vi "S2C_UNITHERM_Proc_CacheState.vi"(7 "Label":string, 8 "Error In":errorcluster, 11 "Data In":string) -> (0 "Error Out":errorcluster, 3 "Data Out":string)   [LabVIEW 2024]
uses:
  S2C_UNITHERM_Proc_Globals.vi
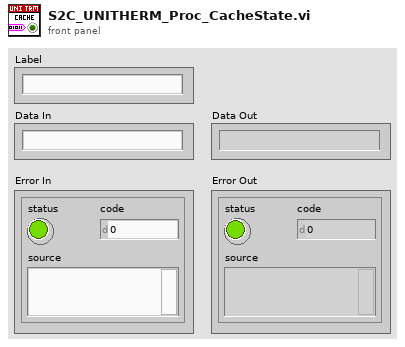
[diagram p1: front panel]
types:
  T1 = cluster{"Resource Name":string, "Baud Rate":u32, "Data Bits":u16, "Parity":u16, "Stop Bits":u16, "Flow Control":u16, "Termination Char":u8, "Enable Termination":bool, "Timeout":u32}
  T2 = cluster{"Resource Name":refnum<visa-resource-name>, "Baud Rate":u32, "Data Bits":u16, "Parity":u16, "Stop Bits":u16, "Flow Control":u16, "Termination Char":u8, "Enable Termination":bool, "Timeout":u32, "P1C1Exe":bool}
  T3 = cluster{"Command":string, "Action":string, "P2C1Exe":bool}
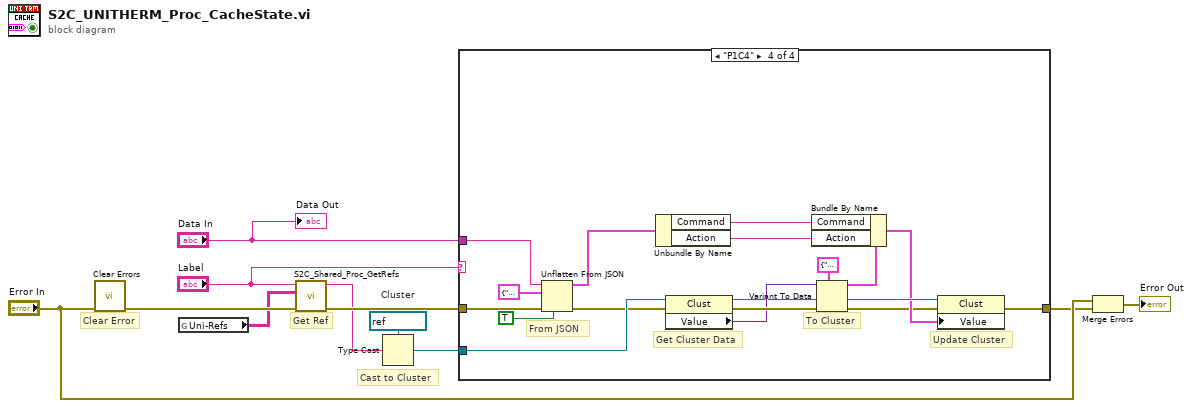
[diagram p0: block diagram]
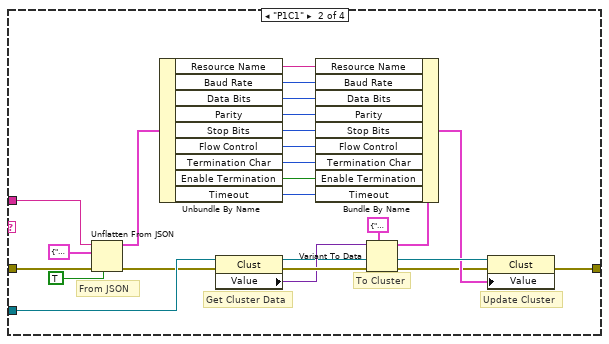
[diagram p3: hidden frame]
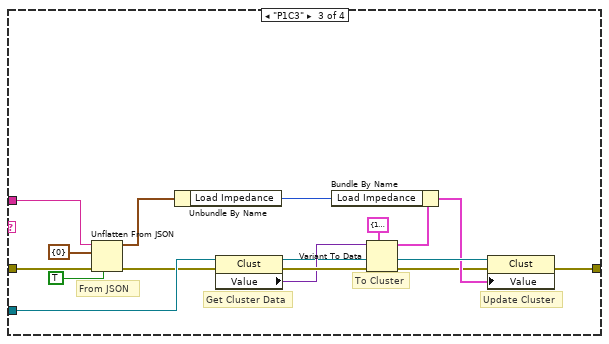
[diagram p4: hidden frame]
diagram:
  w7 = refnum<vi> refnum  # Cluster
  # "Cast to Cluster"
  # "Get Ref"
  # "Clear Error"
  n1 = call <vilib>:"Clear Errors.vi"("error in (no error)"="Error In") -> ("error out"=w4:errorcluster)  [unwired: 5 in, 1 out]
  n2 = global read "S2C_UNITHERM_Proc_Globals.vi" "Uni-Refs"() -> (w1:string[][])
  n3 = call "S2C_Shared_Proc_GetRefs.vi"("Error In"=w4, "Refs"=w1, "Label"="Label") -> ("Error Out"=w9:errorcluster, "Reference"=w6:string)  [unwired: 7 in]
  n4 = Type Cast(type=w7, x=w6) -> (*(type *) &x=w5:refnum<vi>)
  n5 = case shown="\"P1C4\"" "Label" {
    tunnel: w9 -> [w12 w20 w46 w62]
    tunnel: [w12 w14 w40 w56] -> w2
    tunnel: w5 -> [_ w23 w48 w64]
    tunnel: "Data In" -> [_ w18 w44 w60]
    frame "Other", Default {
    }
    frame "P1C1" {
      # "Update Cluster"
      # "To Cluster"
      # "Get Cluster Data"
      # "From JSON"
      n6 = Unflatten From JSON(JSON string=w18, type and defaults=T1 {"Resource Name"="", "Baud Rate"=0, "Data Bits"=5, "Parity"=0, "Stop Bits"=10, "Flow Control"=0, "Termination Char"=0, "Enable Termination"=FALSE, "Timeout"=0}, default null elements? (F)=TRUE, error in (no error)=w20) -> (value=w19:T1, error out=w17:errorcluster)  [unwired: 3 in]
      n7 = Unbundle By Name(w19) -> ("Resource Name"=w32:string, "Baud Rate"=w31:u32, "Data Bits"=w30:u16, "Parity"=w29:u16, "Stop Bits"=w28:u16, "Flow Control"=w27:u16, "Termination Char"=w26:u8, "Enable Termination"=w25:bool, "Timeout"=w24:u32)
      n8 = property class="Clust"(reference=w23, error in=w17) -> (reference out=w16:refnum<vi>, error out=w36:errorcluster, "Value"=w34:variant)
      n9 = Variant To Data(error in=w36, type=T2 {"Resource Name"="", "Baud Rate"=0, "Data Bits"=5, "Parity"=0, "Stop Bits"=10, "Flow Control"=0, "Termination Char"=0, "Enable Termination"=FALSE, "Timeout"=0, "P1C1Exe"=FALSE} ("P1C1"), Variant=w34) -> (data=w33:T2, error out=w13:errorcluster)
      n10 = Bundle By Name(cluster=w33, "Resource Name"=w32, "Baud Rate"=w31, "Data Bits"=w30, "Parity"=w29, "Stop Bits"=w28, "Flow Control"=w27, "Termination Char"=w26, "Enable Termination"=w25, "Timeout"=w24) -> (w15:T2)
      n11 = property class="Clust"(reference=w16, error in=w13, "Value"=w15) -> (error out=w14:errorcluster)  [unwired: 1 out]
    }
    frame "P1C3" {
      # "Update Cluster"
      # "To Cluster"
      # "Get Cluster Data"
      # "From JSON"
      n12 = Unflatten From JSON(JSON string=w44, type and defaults=cluster{"Load Impedance":i32} {"Load Impedance"=0}, default null elements? (F)=TRUE, error in (no error)=w46) -> (value=w45:cluster{"Load Impedance":i32}, error out=w43:errorcluster)  [unwired: 3 in]
      n13 = Unbundle By Name(w45) -> ("Load Impedance"=w49:i32)
      n14 = property class="Clust"(reference=w48, error in=w43) -> (reference out=w42:refnum<vi>, error out=w52:errorcluster, "Value"=w51:variant)
      n15 = Variant To Data(error in=w52, type=cluster{"Load Impedance":i32, "P2C2Exe":bool} {"Load Impedance"=101, "P2C2Exe"=FALSE} ("P2C2"), Variant=w51) -> (data=w50:cluster{"Load Impedance":i32, "P2C2Exe":bool}, error out=w39:errorcluster)
      n16 = Bundle By Name(cluster=w50, "Load Impedance"=w49) -> (w41:cluster{"Load Impedance":i32, "P2C2Exe":bool})
      n17 = property class="Clust"(reference=w42, error in=w39, "Value"=w41) -> (error out=w40:errorcluster)  [unwired: 1 out]
    }
    frame "P1C4" {
      # "Update Cluster"
      # "To Cluster"
      # "Get Cluster Data"
      # "From JSON"
      n18 = Unflatten From JSON(JSON string=w60, type and defaults=cluster{"Command":string, "Action":string} {"Command"="", "Action"=""}, default null elements? (F)=TRUE, error in (no error)=w62) -> (value=w61:cluster{"Command":string, "Action":string}, error out=w59:errorcluster)  [unwired: 3 in]
      n19 = Unbundle By Name(w61) -> ("Command"=w66:string, "Action"=w65:string)
      n20 = property class="Clust"(reference=w64, error in=w59) -> (reference out=w58:refnum<vi>, error out=w69:errorcluster, "Value"=w68:variant)
      n21 = Variant To Data(error in=w69, type=T3 {"Command"="", "Action"="READ", "P2C1Exe"=FALSE} ("P2C1"), Variant=w68) -> (data=w67:T3, error out=w55:errorcluster)
      n22 = Bundle By Name(cluster=w67, "Command"=w66, "Action"=w65) -> (w57:T3)
      n23 = property class="Clust"(reference=w58, error in=w55, "Value"=w57) -> (error out=w56:errorcluster)  [unwired: 1 out]
    }
  }
  n24 = Merge Errors("Error In", w2) -> (→"Error Out":errorcluster)
  "Data Out" <- "Data In"
